vi "PFI-28000-Base_Send Command.vi"(0 "PFI-28000-Base in":refnum<class "PFI-28000-Base.lvclass">, 5 "Command":string, 11 "error in (no error)":errorcluster) -> (4 "PFI-28000-Base out":refnum<class "PFI-28000-Base.lvclass">, 15 "error out":errorcluster)   [LabVIEW 2017, in "PFI-28000-Base.lvclass"]
uses:
  PFI-28000-Base.lvclass
  Utilities/PFI-28000-Utils.lvlib
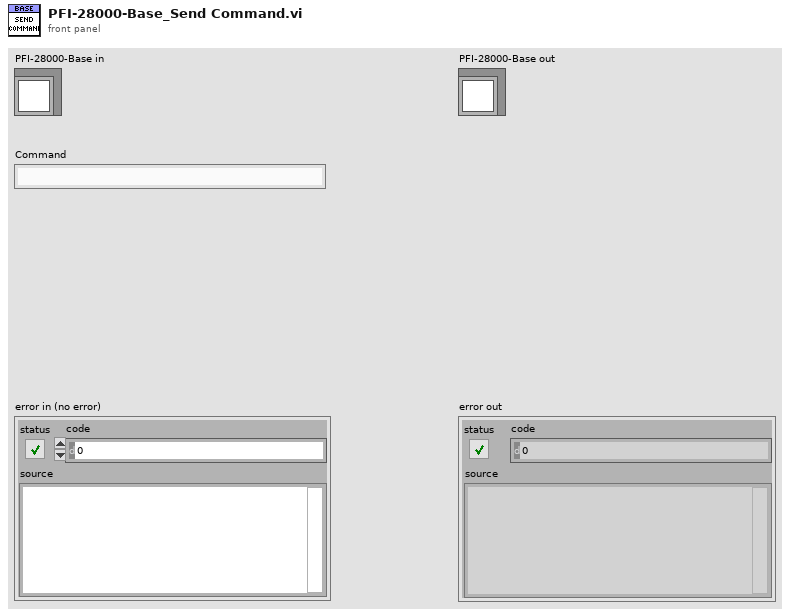
[diagram p1: front panel]
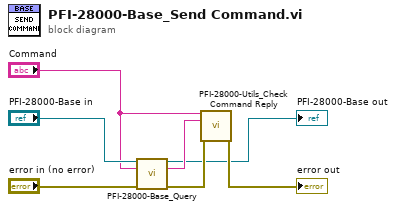
[diagram p0: block diagram]
diagram:
  n1 = call-dynamic "PFI-28000-Base_Query.vi"("PFI-28000-Base in"="PFI-28000-Base in", "Command"="Command", "error in (no error)"="error in (no error)") -> ("PFI-28000-Base out"=→"PFI-28000-Base out":refnum<class "PFI-28000-Base.lvclass">, "Response"=w5:string, "error out"=w3:errorcluster)  [unwired: 9 in, 1 out]
  n2 = call "PFI-28000-Utils_Check Command Reply.vi"("Command"="Command", "Reply"=w5, "error in (no error)"=w3) -> ("error out"=→"error out":errorcluster)  [unwired: 12 in]
